vi "Modified LabVIEW pid controll.vi"(6 "reinitialize? (F)":bool, 7 "output range":cluster{"output high":dbl, "output low":dbl}={"output high"=100.0, "output low"=-100.0} {"output low" format="%.2f"; "output high" format="%.2f"}, 8 "dt (s)":dbl=-1.0 format="%.3f", 9 "PID gains":T1={"proportional gain (Kc)"=1.0, "integral time (Ti, min)"=0.01, "derivative time (Td, min)"=0.0} {"derivative time (Td, min)" format="%.3f"; "integral time (Ti, min)" format="%.3f"; "proportional gain (Kc)" format="%.3f"}, 10 "process variable":dbl format="%.2f", 11 "setpoint":dbl format="%.2f") -> (0 "derivative":dbl, 1 "integrated":dbl, 2 "proportional":dbl, 3 "output":dbl format="%.2f", 4 "dt out (s)":dbl format="%.3f")   [LabVIEW 2020]
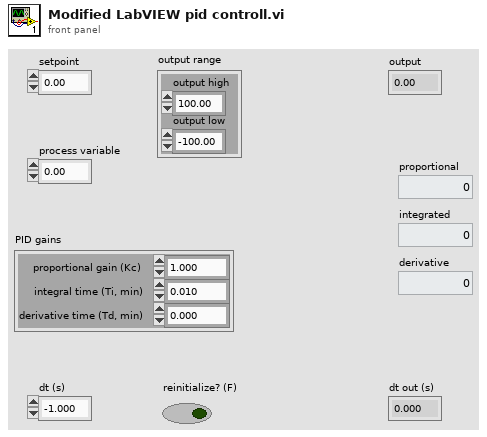
[diagram p1: front panel]
types:
  T1 = cluster{"proportional gain (Kc)":dbl, "integral time (Ti, min)":dbl, "derivative time (Td, min)":dbl}
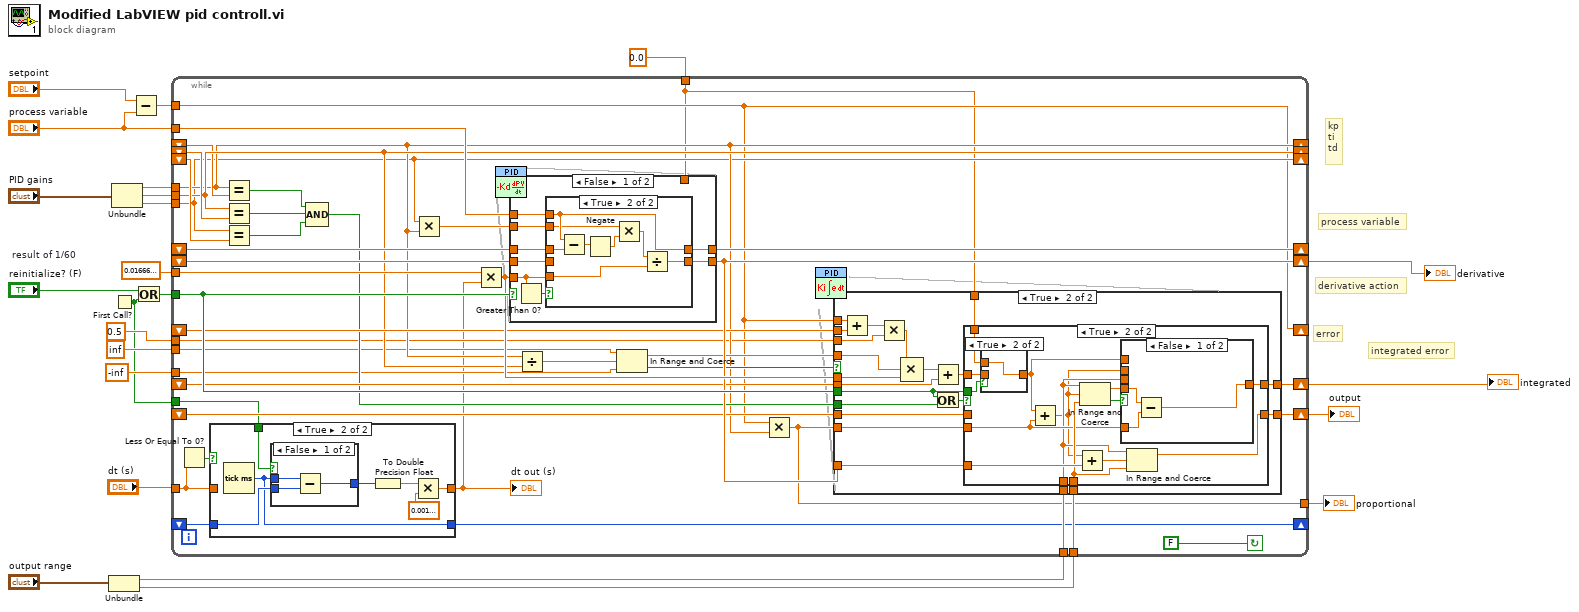
[diagram p0: block diagram]
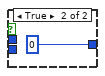
[diagram p3: hidden frame]
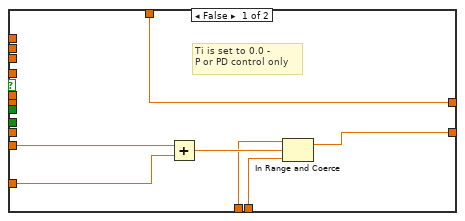
[diagram p4: hidden frame]
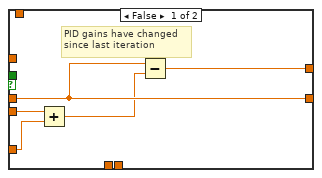
[diagram p5: hidden frame]
diagram:
  w17 = 0.016666666666666666  # result of 1/60
  # "derivative action"
  # "process variable"
  # "kp\nti\ntd"
  # "error"
  # "integrated error"
  n1 = Unbundle("output range") -> ("output high"=w19:dbl, "output low"=w18:dbl)
  n2 = First Call?() -> (First Call?: T/F=w4:bool)
  n3 = Unbundle("PID gains") -> ("proportional gain (Kc)"=w22:dbl, "integral time (Ti, min)"=w21:dbl, "derivative time (Td, min)"=w20:dbl)
  n4 = Subtract(x="setpoint", y="process variable") -> (x-y=w6:dbl)
  n5 = Or(x="reinitialize? (F)", y=w4) -> (x .or. y?=w23:bool)
  n6 = while {
    tunnel: w23 -> [w65]
    shift-left: _ -> [w28]
    shift-right: [w29] -> _
    shift-right: [w38] -> _
    shift-left: _ -> [w39]
    shift-right: [w40] -> _
    shift-left: _ -> [w62]
    shift-right: [w33] -> _
    shift-left: _ -> [w63]
    tunnel: w22 -> [w38]
    tunnel: w21 -> [w40]
    tunnel: w20 -> [w33]
    tunnel: "dt (s)" -> [w27]
    tunnel: w19 -> [w58]
    tunnel: w18 -> [w57]
    tunnel: "process variable" -> [w56]
    shift-right: [w55] -> _
    shift-left: _ -> [w54]
    shift-right: [w53] -> w2
    shift-left: _ -> [w45]
    shift-right: [w52] -> w10
    shift-left: _ -> [w51]
    shift-right: [w32] -> _
    shift-left: _ -> [w50]
    shift-right: [w49] -> w3
    shift-left: _ -> [w48]
    tunnel: w17 -> [w42]
    tunnel: 0.5 ("y") -> [w37]
    tunnel: inf ("upper limit") -> [w35]
    tunnel: -inf ("lower limit") -> [w36]
    tunnel: w6 -> [w32]
    tunnel: 0.0 -> [w31]
    tunnel: w4 -> [w25]
    tunnel: [w24] -> w1
    stop <- FALSE continue-if-true
    n7 = Less Or Equal To 0?(x=w27) -> (x <= 0?=w26:bool)
    n8 = case shown="True" w26 {
      tunnel: [w67 w71] -> w30
      tunnel: w28 -> [w66 w70]
      tunnel: [w66 w69] -> w29
      tunnel: w27 -> [w67 _]
      tunnel: w25 -> [_ w68]
      frame False {
      }
      frame True {
        n9 = Tick Count (ms)() -> (millisecond timer value=w69:u32)
        n10 = case shown="False" w68 {
          tunnel: [w77 u32 0] -> w73
          tunnel: w70 -> [w76 _]
          tunnel: w69 -> [w75 _]
          frame False {
            n11 = Subtract(x=w75, y=w76) -> (x-y=w77:u32)
          }
          frame True {
          }
        }
        n12 = To Double Precision Float(number=w73) -> (double precision float=w72:dbl)
        n13 = Multiply(x=w72, y=0.0010000000474974513) -> (x*y=w71:dbl)
      }
    }
    "dt out (s)" <- w30
    n14 = Equal?(x=w38, y=w39) -> (x = y?=w60:bool)
    n15 = Equal?(x=w40, y=w62) -> (x = y?=w59:bool)
    n16 = Equal?(x=w33, y=w63) -> (x = y?=w61:bool)
    n17 = Compound Arithmetic op=AND(w60, w59, w61) -> (w41:bool)
    n18 = Multiply(x=w33, y=w38) -> (x*y=w44:dbl)
    n19 = Multiply(x=w42, y=w30) -> (x*y=w64:dbl)
    n20 = case shown="False" w65 {
      tunnel: w54 -> [w139 _]
      tunnel: w44 -> [w136 _]
      tunnel: w56 -> [w138 w151]
      tunnel: [w135 w151] -> w55
      tunnel: [w137 w150] -> w53
      tunnel: w45 -> [w133 _]
      tunnel: w64 -> [w132 _]
      tunnel: w31 -> [_ w150]
      frame False {
        n21 = Greater Than 0?(x=w132) -> (x > 0?=w134:bool)
        n22 = case shown="True" w134 {
          tunnel: w139 -> [w141 w147]
          tunnel: w132 -> [_ w146]
          tunnel: w138 -> [_ w144]
          tunnel: [w140 w145] -> w137
          tunnel: w136 -> [_ w142]
          tunnel: [w141 w144] -> w135
          tunnel: w133 -> [w140 _]
          frame False {
            # "dt = 0 min"
          }
          frame True {
            n23 = Subtract(x=w144, y=w147) -> (x-y=w149:dbl)
            n24 = Negate(x=w149) -> (-x=w143:dbl)
            n25 = Multiply(x=w142, y=w143) -> (x*y=w148:dbl)
            n26 = Divide(x=w148, y=w146) -> (x/y=w145:dbl)
          }
        }
      }
      frame True {
      }
    }
    n27 = Divide(x=w38, y=w40) -> (x/y=w43:dbl)
    n28 = In Range and Coerce(upper limit=w35, x=w43, lower limit=w36) -> (coerced(x)=w47:dbl, In Range?=w46:bool)
    n29 = Multiply(x=w32, y=w38) -> (x*y=w24:dbl)
    n30 = case shown="True" w46 {
      tunnel: w32 -> [_ w105]
      tunnel: w50 -> [_ w106]
      tunnel: w48 -> [_ w101]
      tunnel: [w79 w96] -> w49
      tunnel: w47 -> [_ w94]
      tunnel: w24 -> [w84 w99]
      tunnel: [w85 w95] -> w52
      tunnel: w51 -> [_ w97]
      tunnel: w53 -> [w83 w93]
      tunnel: w65 -> [_ w92]
      tunnel: w41 -> [_ w91]
      tunnel: w64 -> [_ w90]
      tunnel: w58 -> [w81 w88]
      tunnel: w57 -> [w80 w89]
      tunnel: w37 -> [_ w87]
      tunnel: w31 -> [w79 w86]
      frame False {
        # "Ti is set to 0.0 -\nP or PD control only"
        n31 = Add(x=w84, y=w83) -> (x+y=w82:dbl)
        n32 = In Range and Coerce(upper limit=w81, x=w82, lower limit=w80) -> (coerced(x)=w85:dbl)  [unwired: 1 out]
      }
      frame True {
        n33 = Add(x=w105, y=w106) -> (x+y=w104:dbl)
        n34 = Multiply(x=w104, y=w87) -> (x*y=w103:dbl)
        n35 = Compound Arithmetic op=MULTIPLY(w103, w94, w90) -> (w102:dbl)
        n36 = Add(x=w102, y=w101) -> (x+y=w100:dbl)
        n37 = Or(x=w92, y=w91) -> (x .or. y?=w98:bool)
        n38 = case shown="True" w98 {
          tunnel: w100 -> [_ w119]
          tunnel: w99 -> [w109 w114]
          tunnel: w97 -> [w111 _]
          tunnel: w92 -> [_ w121]
          tunnel: [w110 w116] -> w96
          tunnel: [w111 w124] -> w95
          tunnel: w93 -> [w108 w123]
          tunnel: w89 -> [_ w122]
          tunnel: w88 -> [_ w113]
          tunnel: w86 -> [_ w120]
          frame False {
            # "PID gains have changed\nsince last iteration"
            n39 = Add(x=w109, y=w108) -> (x+y=w107:dbl)
            n40 = Subtract(x=w111, y=w107) -> (x-y=w110:dbl)
          }
          frame True {
            n41 = case shown="True" w121 {
              tunnel: w120 -> [_ w131]
              tunnel: [w130 w131] -> w118
              tunnel: w119 -> [w130 _]
              frame False {
              }
              frame True {
              }
            }
            n42 = Add(x=w118, y=w114) -> (x+y=w112:dbl)
            n43 = Add(x=w112, y=w123) -> (x+y=w125:dbl)
            n44 = In Range and Coerce(upper limit=w113, x=w112, lower limit=w122) -> (coerced(x)=w115:dbl, In Range?=w117:bool)
            n45 = case shown="False" w117 {
              tunnel: w118 -> [_ w129]
              tunnel: [w126 w129] -> w116
              tunnel: w115 -> [w128 _]
              tunnel: w114 -> [w127 _]
              tunnel: w113 -> [_ _]
              tunnel: w112 -> [_ _]
              frame False {
                n46 = Subtract(x=w128, y=w127) -> (x-y=w126:dbl)
              }
              frame True {
              }
            }
            n47 = In Range and Coerce(upper limit=w113, x=w125, lower limit=w122) -> (coerced(x)=w124:dbl)  [unwired: 1 out]
          }
        }
      }
    }
  }
  "output" <- w10
  "integrated" <- w3
  "derivative" <- w2
  "proportional" <- w1
